vi "editDetails.vi"(8 "error in (no error)":errorcluster, 10 "details":T2, 11 "reference in":refnum<class "Devices Controller.lvclass">) -> (0 "error out":errorcluster, 3 "reference out":refnum<class "Devices Controller.lvclass">)   [LabVIEW 2015, in "Devices Controller.lvclass"]
uses:
  Devices Controller.lvclass
  deviceType.ctl
  APP/excelFile_class/fileType.ctl
  APP/k4b2_class/k4b2.lvclass
  APP/fitmate_class/fitmate.lvclass
  APP/excelFile_class/excelFile.lvclass
  File Controller_llb/File Controller.lvclass
  APP/cpet_class/cpet.lvclass
  APP/rmr_class/rmr.lvclass
  APP/bodpod_class/bodpod.lvclass
  APP/peapod_class/peapod.lvclass
  APP/k5_class/k5.lvclass
  APP/bb-pft_class/bb-pft.lvclass
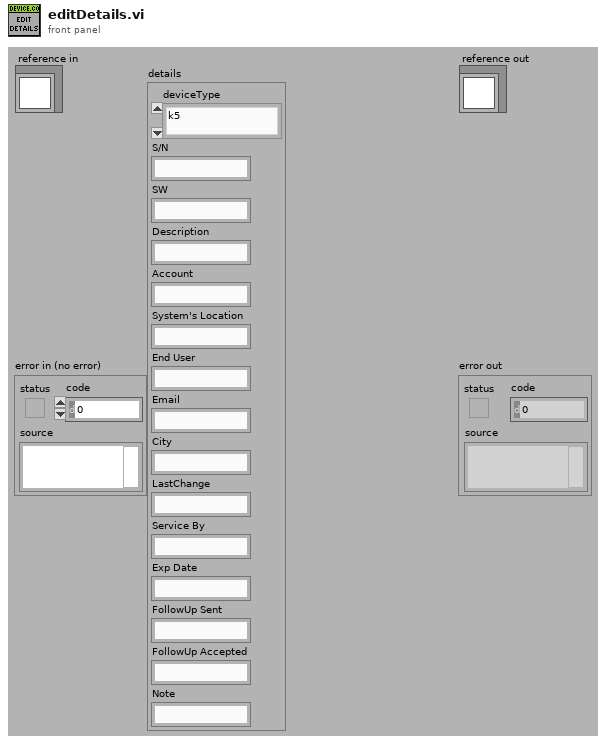
[diagram p1: front panel]
types:
  T1 = typedef "Devices Controller.lvclass/deviceType.ctl" = enum16{"k5", "k4b2", "fitmate", "cpet", "rmr", "bodyBoxPft", "bp", "pp"}
  T2 = cluster{"deviceType":T1, "S/N":string, "SW":string, "Description":string, "Account":string, "System's Location":string, "End User":string, "Email":string, "City":string, "LastChange":string, "Service By":string, "Exp Date":string, "FollowUp Sent":string, "FollowUp Accepted":string, "Note":string}
  T3 = typedef "excelFile.lvclass/fileType.ctl" = enum16{"devices", "items", "partsTracking"}
  T4 = cluster{"deviceType":T1, "S/N":string, "SW":string, "Description":string, "Account":string, "System's Location":string, "End User":string, "Email":string, "City":string, "FollowUp Sent":string, "FollowUp Accepted":string, "Note":string}
  T5 = typedef "Devices Controller.lvclass/ObjectAttributesRef.ctl" = refnum<data-value>
  T6 = typedef "Devices Controller.lvclass/ObjectAttributes.ctl" = cluster{"MyAttribute":dbl, "file_controller_ref":refnum<class "File Controller.lvclass">, "data":string[][][], "devices_refs":cluster{"k4b2_refs":refnum<class "k4b2.lvclass">[], "rmr_refs":refnum<class "rmr.lvclass">[], "bod_pod_refs":refnum<class "bodpod.lvclass">[], "cpet_refs":refnum<class "cpet.lvclass">[], "fitmate_refs":refnum<class "fitmate.lvclass">[], "pea_pod_refs":refnum<class "peapod.lvclass">[], "k5_refs":refnum<class "k5.lvclass">[], "bb-pft_refs":refnum<class "bb-pft.lvclass">[]}}
  T7 = cluster{"k4b2_refs":refnum<class "k4b2.lvclass">[], "rmr_refs":refnum<class "rmr.lvclass">[], "bod_pod_refs":refnum<class "bodpod.lvclass">[], "cpet_refs":refnum<class "cpet.lvclass">[], "fitmate_refs":refnum<class "fitmate.lvclass">[], "pea_pod_refs":refnum<class "peapod.lvclass">[], "k5_refs":refnum<class "k5.lvclass">[], "bb-pft_refs":refnum<class "bb-pft.lvclass">[]}
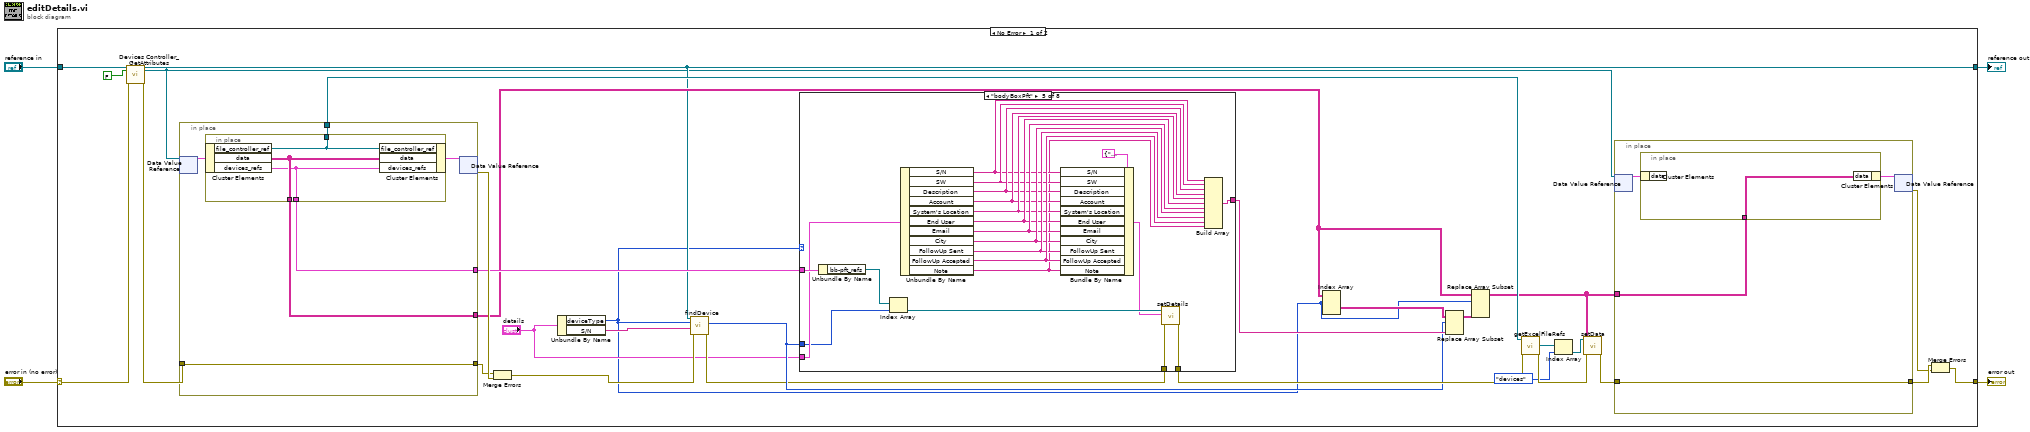
[diagram p0: block diagram]
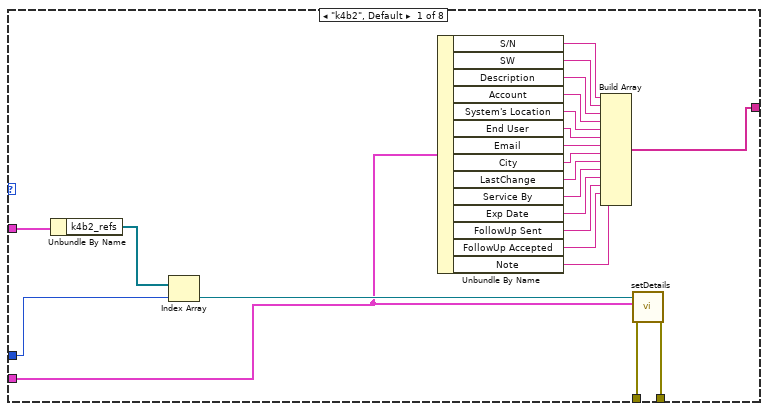
[diagram p2: hidden frame]
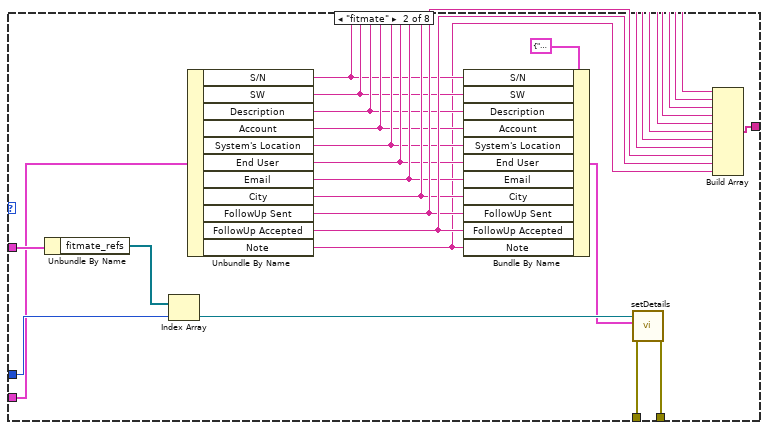
[diagram p3: hidden frame]
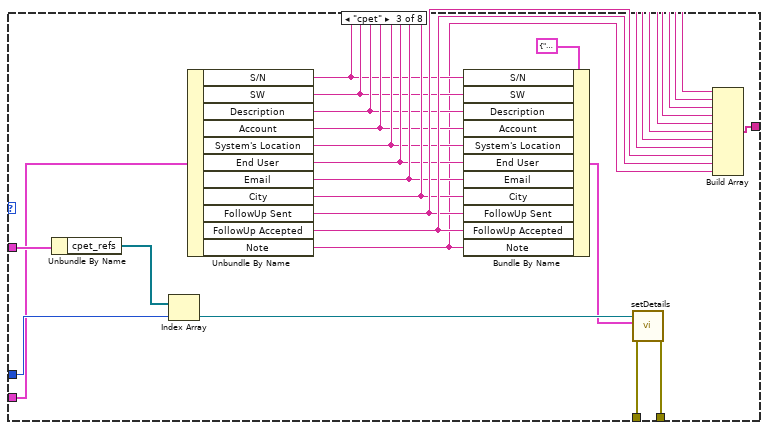
[diagram p4: hidden frame]
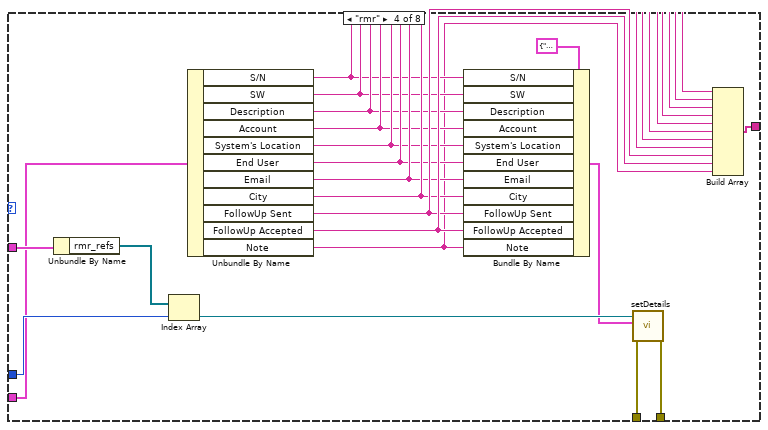
[diagram p5: hidden frame]
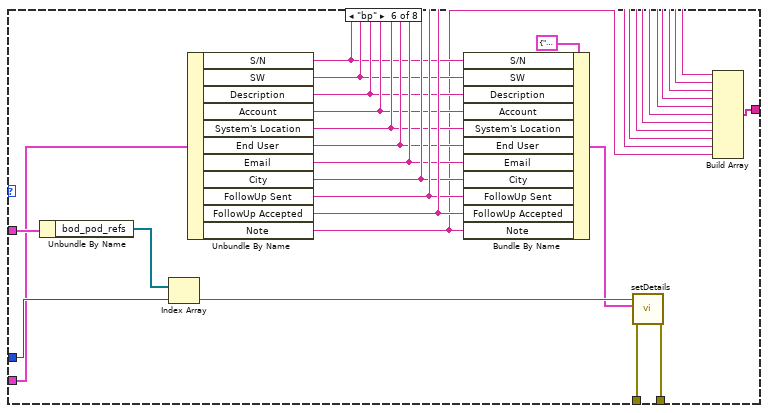
[diagram p6: hidden frame]
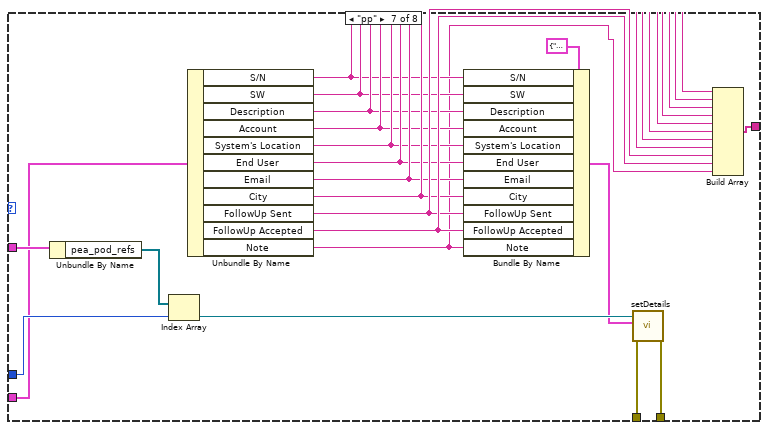
[diagram p7: hidden frame]
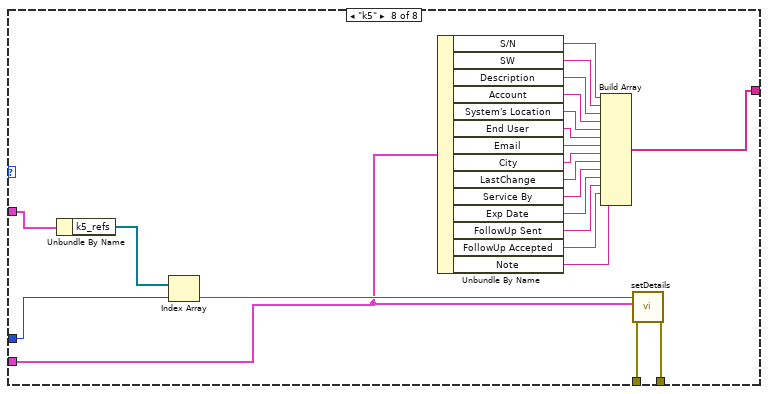
[diagram p8: hidden frame]
diagram:
  n1 = case shown="No Error" "error in (no error)" {
    selector: "error in (no error)" -> [w30 w220]
    tunnel: [w7 w220] -> w3
    tunnel: [w13 w219] -> w1
    tunnel: "reference in" -> [w32 w219]
    frame No Error {
      n2 = call "Devices Controller_GetAttributes.vi"("reference in"=w32, "return data? (T)"=FALSE, "error in (no error)"=w30) -> ("reference out"=w13:refnum<class "Devices Controller.lvclass">, "attributes ref"=w9:T5, "error out"=w29:errorcluster)  [unwired: 13 in, 1 out]
      n3 = in-place {
        in-place-border: w29 -> [w213]
        in-place-border: [w213] -> w33
        in-place-border: [w212] -> w20
        in-place-border: [w211] -> w28
        in-place-border: [w210] -> w18
        n4 = in-place-dvr #1(w9) -> (w214:T6)  [unwired: 1 out]
        n5 = in-place {
          in-place-border: [w218] -> w212
          in-place-border: [w217] -> w211
          in-place-border: [w216] -> w210
          n6 = in-place-cluster #2(w214) -> ("file_controller_ref"=w216:refnum<class "File Controller.lvclass">, "data"=w218:string[][][], "devices_refs"=w217:T7)
          n7 = in-place-cluster #2("file_controller_ref"=w216, "data"=w218, "devices_refs"=w217) -> (w215:T6)
        }
        n8 = in-place-dvr #1(w215) -> (w34:errorcluster)  [unwired: 1 out]
      }
      n9 = Merge Errors(w33, w34) -> (w15:errorcluster)
      n10 = Unbundle By Name("details") -> ("deviceType"=w5:T1, "S/N"=w17:string)
      n11 = call "findDevice.vi"("error in (no error)"=w15, "S/N:"=w17, "Device Type:"=w5, "reference in"=w13) -> ("error out"=w14:errorcluster, "index of element"=w16:i32)  [unwired: 4 in, 2 out]
      n12 = case shown="\"bodyBoxPft\"" w5 {
        tunnel: w28 -> [w61 w82 w103 w124 w130 w166 w187 w193]
        tunnel: w16 -> [w57 w78 w99 w120 w128 w162 w183 w189]
        tunnel: w14 -> [w60 w81 w102 w123 w127 w165 w186 w192]
        tunnel: [w59 w80 w101 w122 w126 w164 w185 w191] -> w21
        tunnel: "details" -> [w41 w76 w97 w118 w129 w160 w181 w188]
        tunnel: [w42 w67 w88 w109 w125 w151 w172 w190] -> w19
        frame "k4b2", Default {
          n13 = Unbundle By Name(w61) -> ("k4b2_refs"=w58:refnum<class "k4b2.lvclass">[])
          n14 = Index Array(array=w58, index=w57) -> (element=w56:refnum<class "k4b2.lvclass">)
          n15 = Unbundle By Name(w41) -> ("S/N"=w55:string, "SW"=w54:string, "Description"=w53:string, "Account"=w52:string, "System's Location"=w51:string, "End User"=w50:string, "Email"=w49:string, "City"=w48:string, "LastChange"=w47:string, "Service By"=w46:string, "Exp Date"=w45:string, "FollowUp Sent"=w44:string, "FollowUp Accepted"=w43:string, "Note"=w40:string)
          n16 = Build Array(w55, w54, w53, w52, w51, w50, w49, w48, w47, w46, w45, w44, w43, w40) -> (w42:string[])
          n17 = call "setDetails.vi"("error in (no error)"=w60, "details"=w41, "reference in"=w56) -> ("error out"=w59:errorcluster)  [unwired: 7 in, 1 out]
        }
        frame "fitmate" {
          n18 = Unbundle By Name(w82) -> ("fitmate_refs"=w79:refnum<class "fitmate.lvclass">[])
          n19 = Index Array(array=w79, index=w78) -> (element=w77:refnum<class "fitmate.lvclass">)
          n20 = Unbundle By Name(w76) -> ("S/N"=w65:string, "SW"=w66:string, "Description"=w68:string, "Account"=w69:string, "System's Location"=w70:string, "End User"=w71:string, "Email"=w72:string, "City"=w73:string, "FollowUp Sent"=w74:string, "FollowUp Accepted"=w75:string, "Note"=w62:string)
          n21 = Bundle By Name(cluster=T4 {"deviceType"=enum."k5", "S/N"="", "SW"="", "Description"="", "Account"="", "System's Location"="", "End User"="", "Email"="", "City"="", "FollowUp Sent"="", "FollowUp Accepted"="", "Note"=""} ("details"), "S/N"=w65, "SW"=w66, "Description"=w68, "Account"=w69, "System's Location"=w70, "End User"=w71, "Email"=w72, "City"=w73, "FollowUp Sent"=w74, "FollowUp Accepted"=w75, "Note"=w62) -> (w63:T4)
          n22 = call "setDetails.vi"("error in (no error)"=w81, "details"=w63, "reference in"=w77) -> ("error out"=w80:errorcluster)  [unwired: 7 in, 1 out]
          n23 = Build Array(w65, w66, w68, w69, w70, w71, w72, w73, w74, w75, w62) -> (w67:string[])
        }
        frame "cpet" {
          n24 = Unbundle By Name(w103) -> ("cpet_refs"=w100:refnum<class "cpet.lvclass">[])
          n25 = Index Array(array=w100, index=w99) -> (element=w98:refnum<class "cpet.lvclass">)
          n26 = Unbundle By Name(w97) -> ("S/N"=w86:string, "SW"=w87:string, "Description"=w89:string, "Account"=w90:string, "System's Location"=w91:string, "End User"=w92:string, "Email"=w93:string, "City"=w94:string, "FollowUp Sent"=w95:string, "FollowUp Accepted"=w96:string, "Note"=w83:string)
          n27 = Bundle By Name(cluster=T4 {"deviceType"=enum."k5", "S/N"="", "SW"="", "Description"="", "Account"="", "System's Location"="", "End User"="", "Email"="", "City"="", "FollowUp Sent"="", "FollowUp Accepted"="", "Note"=""} ("details"), "S/N"=w86, "SW"=w87, "Description"=w89, "Account"=w90, "System's Location"=w91, "End User"=w92, "Email"=w93, "City"=w94, "FollowUp Sent"=w95, "FollowUp Accepted"=w96, "Note"=w83) -> (w84:T4)
          n28 = call "setDetails.vi"("error in (no error)"=w102, "details"=w84, "reference in"=w98) -> ("error out"=w101:errorcluster)  [unwired: 7 in, 1 out]
          n29 = Build Array(w86, w87, w89, w90, w91, w92, w93, w94, w95, w96, w83) -> (w88:string[])
        }
        frame "rmr" {
          n30 = Unbundle By Name(w124) -> ("rmr_refs"=w121:refnum<class "rmr.lvclass">[])
          n31 = Index Array(array=w121, index=w120) -> (element=w119:refnum<class "rmr.lvclass">)
          n32 = Unbundle By Name(w118) -> ("S/N"=w107:string, "SW"=w108:string, "Description"=w110:string, "Account"=w111:string, "System's Location"=w112:string, "End User"=w113:string, "Email"=w114:string, "City"=w115:string, "FollowUp Sent"=w116:string, "FollowUp Accepted"=w117:string, "Note"=w104:string)
          n33 = Bundle By Name(cluster=T4 {"deviceType"=enum."k5", "S/N"="", "SW"="", "Description"="", "Account"="", "System's Location"="", "End User"="", "Email"="", "City"="", "FollowUp Sent"="", "FollowUp Accepted"="", "Note"=""} ("details"), "S/N"=w107, "SW"=w108, "Description"=w110, "Account"=w111, "System's Location"=w112, "End User"=w113, "Email"=w114, "City"=w115, "FollowUp Sent"=w116, "FollowUp Accepted"=w117, "Note"=w104) -> (w105:T4)
          n34 = call "setDetails.vi"("error in (no error)"=w123, "details"=w105, "reference in"=w119) -> ("error out"=w122:errorcluster)  [unwired: 7 in, 1 out]
          n35 = Build Array(w107, w108, w110, w111, w112, w113, w114, w115, w116, w117, w104) -> (w109:string[])
        }
        frame "bodyBoxPft" {
          n36 = Unbundle By Name(w130) -> ("bb-pft_refs"=w145:refnum<class "bb-pft.lvclass">[])
          n37 = Index Array(array=w145, index=w128) -> (element=w144:refnum<class "bb-pft.lvclass">)
          n38 = Unbundle By Name(w129) -> ("S/N"=w134:string, "SW"=w135:string, "Description"=w136:string, "Account"=w137:string, "System's Location"=w138:string, "End User"=w139:string, "Email"=w140:string, "City"=w141:string, "FollowUp Sent"=w142:string, "FollowUp Accepted"=w143:string, "Note"=w131:string)
          n39 = Bundle By Name(cluster=T4 {"deviceType"=enum."k5", "S/N"="", "SW"="", "Description"="", "Account"="", "System's Location"="", "End User"="", "Email"="", "City"="", "FollowUp Sent"="", "FollowUp Accepted"="", "Note"=""} ("details"), "S/N"=w134, "SW"=w135, "Description"=w136, "Account"=w137, "System's Location"=w138, "End User"=w139, "Email"=w140, "City"=w141, "FollowUp Sent"=w142, "FollowUp Accepted"=w143, "Note"=w131) -> (w132:T4)
          n40 = call "setDetails.vi"("error in (no error)"=w127, "details"=w132, "reference in"=w144) -> ("error out"=w126:errorcluster)  [unwired: 7 in, 1 out]
          n41 = Build Array(w134, w135, w136, w137, w138, w139, w140, w141, w142, w143, w131) -> (w125:string[])
        }
        frame "bp" {
          n42 = Unbundle By Name(w166) -> ("bod_pod_refs"=w163:refnum<class "bodpod.lvclass">[])
          n43 = Index Array(array=w163, index=w162) -> (element=w161:refnum<class "bodpod.lvclass">)
          n44 = Unbundle By Name(w160) -> ("S/N"=w149:string, "SW"=w150:string, "Description"=w152:string, "Account"=w153:string, "System's Location"=w154:string, "End User"=w155:string, "Email"=w156:string, "City"=w157:string, "FollowUp Sent"=w158:string, "FollowUp Accepted"=w159:string, "Note"=w147:string)
          n45 = Bundle By Name(cluster=T4 {"deviceType"=enum."k5", "S/N"="", "SW"="", "Description"="", "Account"="", "System's Location"="", "End User"="", "Email"="", "City"="", "FollowUp Sent"="", "FollowUp Accepted"="", "Note"=""} ("details"), "S/N"=w149, "SW"=w150, "Description"=w152, "Account"=w153, "System's Location"=w154, "End User"=w155, "Email"=w156, "City"=w157, "FollowUp Sent"=w158, "FollowUp Accepted"=w159, "Note"=w147) -> (w146:T4)
          n46 = call "setDetails.vi"("error in (no error)"=w165, "details"=w146, "reference in"=w161) -> ("error out"=w164:errorcluster)  [unwired: 7 in, 1 out]
          n47 = Build Array(w149, w150, w152, w153, w154, w155, w156, w157, w158, w159, w147) -> (w151:string[])
        }
        frame "pp" {
          n48 = Unbundle By Name(w187) -> ("pea_pod_refs"=w184:refnum<class "peapod.lvclass">[])
          n49 = Index Array(array=w184, index=w183) -> (element=w182:refnum<class "peapod.lvclass">)
          n50 = Unbundle By Name(w181) -> ("S/N"=w170:string, "SW"=w171:string, "Description"=w173:string, "Account"=w174:string, "System's Location"=w175:string, "End User"=w176:string, "Email"=w177:string, "City"=w178:string, "FollowUp Sent"=w179:string, "FollowUp Accepted"=w180:string, "Note"=w167:string)
          n51 = Bundle By Name(cluster=T4 {"deviceType"=enum."k5", "S/N"="", "SW"="", "Description"="", "Account"="", "System's Location"="", "End User"="", "Email"="", "City"="", "FollowUp Sent"="", "FollowUp Accepted"="", "Note"=""} ("details"), "S/N"=w170, "SW"=w171, "Description"=w173, "Account"=w174, "System's Location"=w175, "End User"=w176, "Email"=w177, "City"=w178, "FollowUp Sent"=w179, "FollowUp Accepted"=w180, "Note"=w167) -> (w168:T4)
          n52 = call "setDetails.vi"("error in (no error)"=w186, "details"=w168, "reference in"=w182) -> ("error out"=w185:errorcluster)  [unwired: 7 in, 1 out]
          n53 = Build Array(w170, w171, w173, w174, w175, w176, w177, w178, w179, w180, w167) -> (w172:string[])
        }
        frame "k5" {
          n54 = Unbundle By Name(w193) -> ("k5_refs"=w209:refnum<class "k5.lvclass">[])
          n55 = Index Array(array=w209, index=w189) -> (element=w208:refnum<class "k5.lvclass">)
          n56 = Unbundle By Name(w188) -> ("S/N"=w207:string, "SW"=w206:string, "Description"=w205:string, "Account"=w204:string, "System's Location"=w203:string, "End User"=w202:string, "Email"=w201:string, "City"=w200:string, "LastChange"=w199:string, "Service By"=w198:string, "Exp Date"=w197:string, "FollowUp Sent"=w196:string, "FollowUp Accepted"=w195:string, "Note"=w194:string)
          n57 = Build Array(w207, w206, w205, w204, w203, w202, w201, w200, w199, w198, w197, w196, w195, w194) -> (w190:string[])
          n58 = call "setDetails.vi"("error in (no error)"=w192, "details"=w188, "reference in"=w208) -> ("error out"=w191:errorcluster)  [unwired: 7 in, 1 out]
        }
      }
      n59 = Index Array(array=w20, index (dim 0)=w5) -> (element=w27:string[][])  [unwired: 2 in]
      n60 = Replace Array Subset(array=w27, new element=w19, index (row)=w16) -> (w26:string[][])  [unwired: 1 in]
      n61 = Replace Array Subset(array=w20, new element=w26, index (dim 0)=w5) -> (w10:string[][][])  [unwired: 2 in]
      n62 = call "getExcelFileRefs.vi"("error in (no error)"=w21, "reference in"=w18) -> ("error out"=w25:errorcluster, "excelFile_refs"=w24:refnum<class "excelFile.lvclass">[])  [unwired: 7 in, 1 out]
      n63 = Index Array(array=w24, index=fileType."devices" ("fileType")) -> (element=w23:refnum<class "excelFile.lvclass">)
      n64 = call "setData.vi"("error in (no error)"=w25, "data"=w10, "reference in"=w23) -> ("error out"=w11:errorcluster)  [unwired: 7 in, 1 out]
      n65 = in-place {
        in-place-border: w11 -> [w36]
        in-place-border: [w36] -> w8
        in-place-border: w10 -> [w35]
        n66 = in-place-dvr #3(w9) -> (w37:T6)  [unwired: 1 out]
        n67 = in-place {
          in-place-border: w35 -> [w39]
          n68 = in-place-cluster #4(w37) -> ()  [unwired: 1 out]
          n69 = in-place-cluster #4("data"=w39) -> (w38:T6)
        }
        n70 = in-place-dvr #3(w38) -> (w6:errorcluster)  [unwired: 1 out]
      }
      n71 = Merge Errors(w8, w6) -> (w7:errorcluster)
    }
    frame Error {
    }
  }
  "error out" <- w3
  "reference out" <- w1
